vi "Validate.vi"(8 "error in (no error)":errorcluster, 9 "in build?":bool, 10 "proj refnum":refnum<vi>, 11 "IB_Source_Build in":refnum<class "IB_Source_Build.lvclass">) -> (0 "error out":errorcluster, 3 "IB_Source_Build out":refnum<class "IB_Source_Build.lvclass">)   [LabVIEW 2020, in "IB_Source_Build.lvclass"]
uses:
  <vilib>/AppBuilder/IB_Classes/Source/Container/Build/IB_Source_Build.lvclass
  <vilib>/AppBuilder/IB_Classes/Source/Container/Build/IB_Source_Build.lvclass/IB_Source_Build.ctl
  <vilib>/AppBuilder/IB_Classes/Source/IB_Source.lvclass
  <vilib>/AppBuilder/IB_Classes/Source/Container/IB_Source_Container.lvclass
  <vilib>/AppBuilder/IB_Classes/Source/File/CtrFile/IB_CtrFile.lvclass
  e:/builds/penguin/labview/branches/2020/dev/dist/vi.lib/AppBuilder/IB_Classes/Source/Container/IB_Source_Container.lvclass
  e:/builds/penguin/labview/branches/2020/dev/dist/vi.lib/AppBuilder/IB_Classes/Source/IB_Source.lvclass
  e:/builds/penguin/labview/branches/2020/dev/dist/vi.lib/AppBuilder/IB_Classes/Source/Container/Build/IB_Source_Build.lvclass
  e:/builds/penguin/labview/branches/2020/dev/dist/vi.lib/AppBuilder/IB_Classes/Source/File/IB_Source_File.lvclass
  e:/builds/penguin/labview/branches/2020/dev/dist/vi.lib/AppBuilder/IB_Classes/Source/File/CtrFile/IB_CtrFile.lvclass
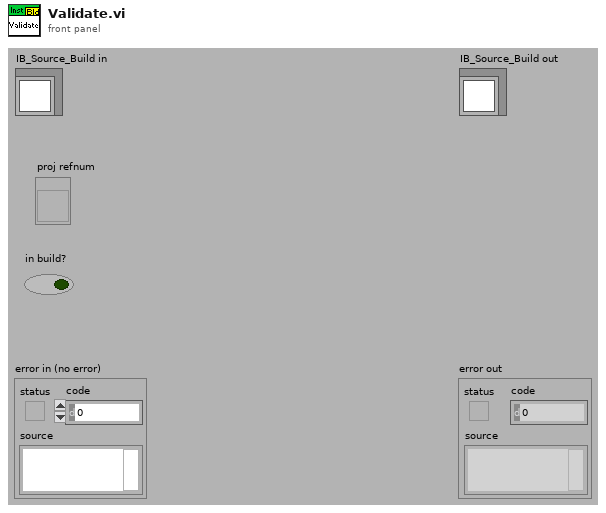
[diagram p1: front panel]
types:
  T1 = typedef "IB_Source_Container.ctl" = cluster{"files":refnum<class "IB_CtrFile.lvclass">[], "previewed?":bool, "preview error?":bool}
  T2 = typedef "IB_Source.ctl" = cluster{"name":string, "sourceTag":string, "destTag":string, "path":path, "eng_installPath":string, "UI_inBuild?":bool, "str ref?":bool}
  T3 = typedef "SRdB_Bld.ctl" = cluster{"ItemID":string, "FileItemIDs":string[], "RelPaths":string[], "AbsPaths":path[], "preview error?":bool, "Dependencies":T4[]}
  T4 = typedef "AB_Dependency.ctl" = cluster{"path":path, "delimited name":string, "type":T5}
  T5 = typedef "NI_FileType.lvlib/LVFileType.ctl" = enum32{"Invalid file", "Unknown type", "Instrument", "Control", "Polymorphic VI", "Project", "Library", "LVClass", "XControl", "XNode", "Shared library", ".NET assembly", "ActiveX interface", "CIN", "Run-time menu", "Palette menu", "Help file", "LLB", "XNode Edit Dependency", "Class Private Data Control", "Statechart", "MathScript .m file", "Ladder Diagram", "LVLibp", "XNode Build Dependency"}
  T6 = typedef "IB_CtrFile.ctl" = cluster{"parentTag":string, "force save?":bool}
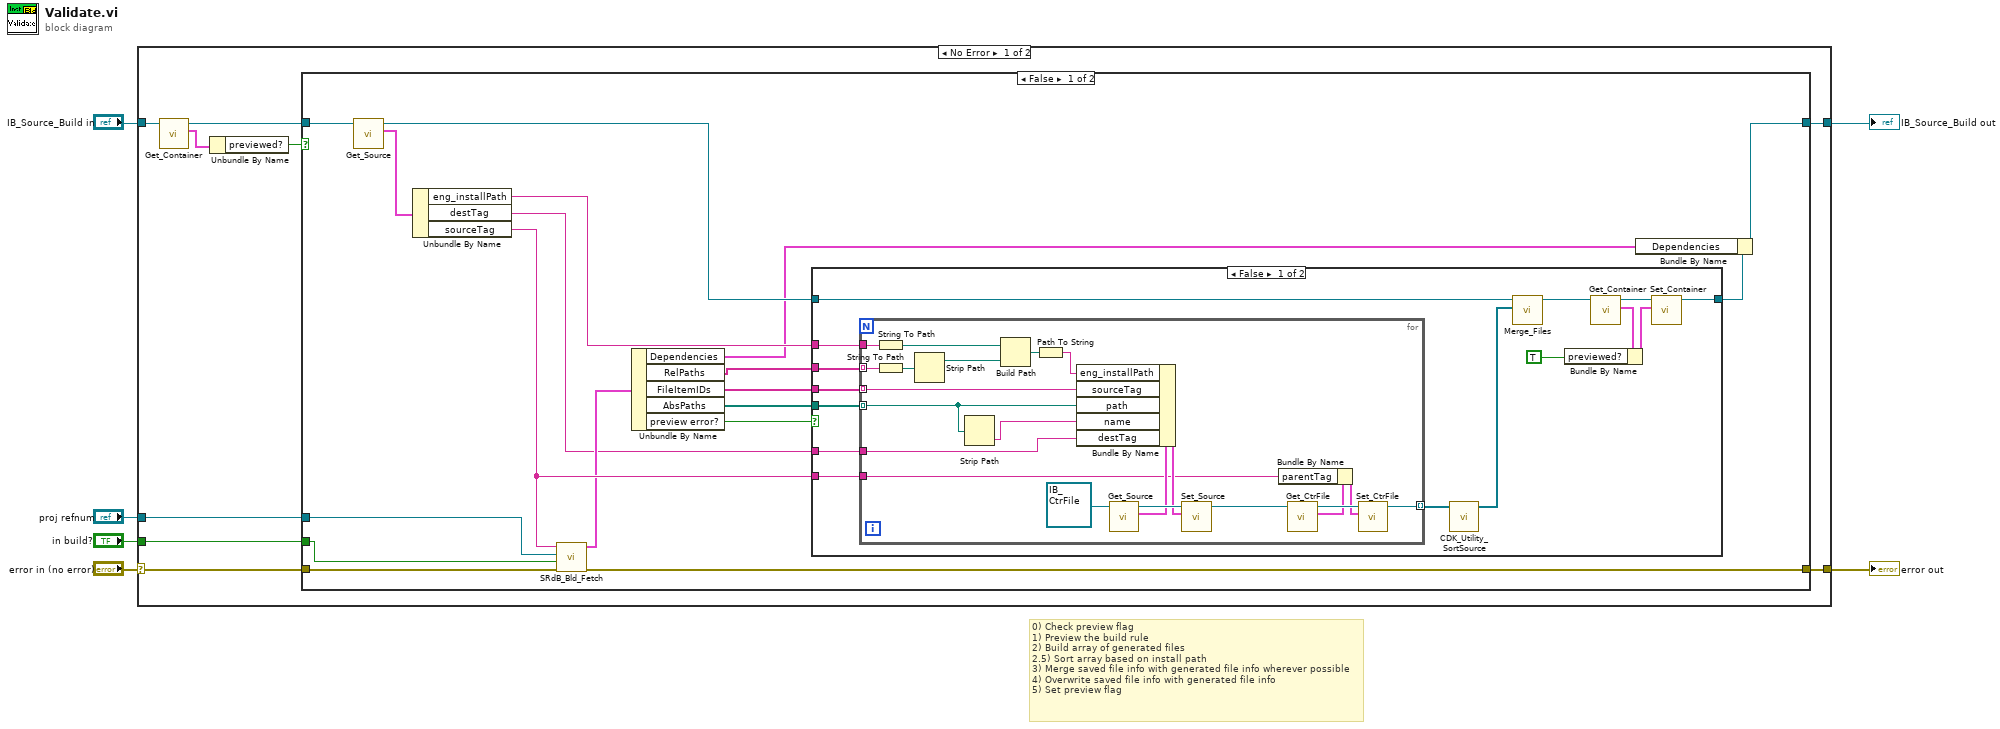
[diagram p0: block diagram]
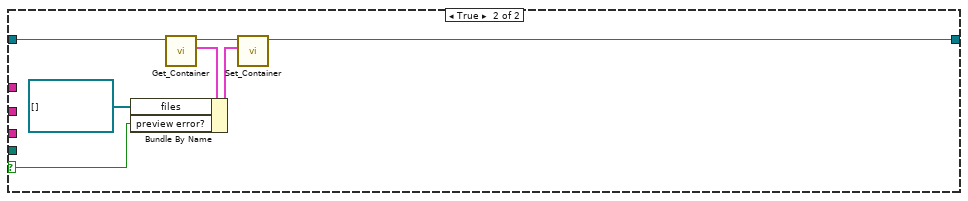
[diagram p2: hidden frame]
diagram:
  # "0) Check preview flag\n1) Preview the build rule\n2) Build array of generated files\n2.5) Sort array based on install path\n3) Merge saved file info with generated file info wherever possible\n4) Overwrite saved file info with generated file info\n5) Set preview flag"
  n1 = case shown="No Error" "error in (no error)" {
    selector: "error in (no error)" -> [w13 w80]
    tunnel: [w12 w80] -> w5
    tunnel: "IB_Source_Build in" -> [w10 w79]
    tunnel: "proj refnum" -> [w14 _]
    tunnel: [w15 w79] -> w2
    tunnel: "in build?" -> [w7 _]
    frame No Error {
      n2 = call <vilib>:"Get_Container.vi"("IB_Source_Container in"=w10) -> ("data"=w8:T1, "IB_Source_Container out"=w9:refnum<class "IB_Source_Build.lvclass">)  [unwired: 1 in, 8 out]
      n3 = Unbundle By Name(w8) -> ("previewed?"=w11:bool)
      n4 = case shown="False" w11 {
        tunnel: w9 -> [w21 w78]
        tunnel: [w18 w78] -> w15
        tunnel: w14 -> [w22 _]
        tunnel: w13 -> [w30 w77]
        tunnel: [w23 w77] -> w12
        tunnel: w7 -> [w19 _]
        frame False {
          n5 = call <vilib>:"Get_Source.vi"("IB_Source in"=w21) -> ("data"=w33:T2, "IB_Source out"=w24:refnum<class "IB_Source_Build.lvclass">)  [unwired: 1 in, 8 out]
          n6 = Unbundle By Name(w33) -> ("eng_installPath"=w32:string, "destTag"=w25:string, "sourceTag"=w31:string)
          n7 = call <resource>:"SRdB_Bld_Fetch.vi"("error in (no error)"=w30, "in build?"=w19, "Project"=w22, "itemID"=w31) -> ("error out"=w23:errorcluster, "build"=w29:T3)  [unwired: 6 out]
          n8 = Unbundle By Name(w29) -> ("Dependencies"=w16:T4[], "RelPaths"=w28:string[], "FileItemIDs"=w27:string[], "AbsPaths"=w26:path[], "preview error?"=w20:bool)
          n9 = case shown="False" w20 {
            selector: w20 -> [_ w70]
            tunnel: w32 -> [w48 _]
            tunnel: [w35 w72] -> w17
            tunnel: w31 -> [w45 _]
            tunnel: w28 -> [w44 _]
            tunnel: w27 -> [w43 _]
            tunnel: w26 -> [w42 _]
            tunnel: w25 -> [w41 _]
            tunnel: w24 -> [w40 w73]
            frame False {
              n10 = for {
                tunnel: w42 -> [w65] mode=indexing
                tunnel: w43 -> [w66] mode=indexing
                tunnel: [w54] -> w47 mode=indexing
                tunnel: w44 -> [w61] mode=indexing
                tunnel: w48 -> [w60]
                tunnel: w41 -> [w56]
                tunnel: w45 -> [w49]
                n11 = String To Path(string=w60) -> (path=w62:path)
                n12 = String To Path(string=w61) -> (path=w58:path)
                n13 = Strip Path(path=w58) -> (stripped path=w57:path)  [unwired: 1 out]
                n14 = Strip Path(path=w65) -> (name=w64:string)  [unwired: 1 out]
                n15 = Build Path(base path=w62, name or relative path=w57) -> (appended path=w63:path)
                n16 = Path To String(path=w63) -> (string=w59:string)
                n17 = call <vilib>:"Get_Source.vi"("IB_Source in"=refnum<class "IB_CtrFile.lvclass"> refnum ("IB_CtrFile.lvclass")) -> ("data"=w68:T2, "IB_Source out"=w69:refnum<class "IB_CtrFile.lvclass">)  [unwired: 1 in, 8 out]
                n18 = Bundle By Name(cluster=w68, "eng_installPath"=w59, "sourceTag"=w66, "path"=w65, "name"=w64, "destTag"=w56) -> (w67:T2)
                n19 = call <vilib>:"Set_Source.vi"("data"=w67, "IB_Source in"=w69) -> ("IB_Source out"=w53:refnum<class "IB_CtrFile.lvclass">)  [unwired: 1 in, 8 out]
                n20 = call <vilib>:"Get_CtrFile.vi"("IB_CtrFile in"=w53) -> ("parentTag"=w51:T6, "IB_CtrFile out"=w52:refnum<class "IB_CtrFile.lvclass">)  [unwired: 1 in, 8 out]
                n21 = Bundle By Name(cluster=w51, "parentTag"=w49) -> (w50:T6)
                n22 = call <vilib>:"Set_CtrFile.vi"("parentTag"=w50, "IB_CtrFile in"=w52) -> ("IB_CtrFile out"=w54:refnum<class "IB_CtrFile.lvclass">)  [unwired: 1 in, 8 out]
              }
              n23 = call <resource>:"CDK_Utility_SortSource.vi"("Source in"=w47) -> ("Source out"=w46:refnum<class "IB_CtrFile.lvclass">[])  [unwired: 10 out]
              n24 = call <vilib>:"Merge_Files.vi"("files"=w46, "IB_Source_Container in"=w40) -> ("IB_Source_Container out"=w36:refnum<class "IB_Source_Build.lvclass">)  [unwired: 2 in, 7 out]
              n25 = call <vilib>:"Get_Container.vi"("IB_Source_Container in"=w36) -> ("data"=w39:T1, "IB_Source_Container out"=w38:refnum<class "IB_Source_Build.lvclass">)  [unwired: 1 in, 8 out]
              n26 = Bundle By Name(cluster=w39, "previewed?"=TRUE) -> (w37:T1)
              n27 = call <vilib>:"Set_Container.vi"("data"=w37, "IB_Source_Container in"=w38) -> ("IB_Source_Container out"=w35:refnum<class "IB_Source_Build.lvclass">)  [unwired: 1 in, 8 out]
            }
            frame True {
              n28 = call <vilib>:"Get_Container.vi"("IB_Source_Container in"=w73) -> ("data"=w76:T1, "IB_Source_Container out"=w75:refnum<class "IB_Source_Build.lvclass">)  [unwired: 1 in, 8 out]
              n29 = Bundle By Name(cluster=w76, "files"=refnum<class "IB_CtrFile.lvclass">[] [], "preview error?"=w70) -> (w74:T1)
              n30 = call <vilib>:"Set_Container.vi"("data"=w74, "IB_Source_Container in"=w75) -> ("IB_Source_Container out"=w72:refnum<class "IB_Source_Build.lvclass">)  [unwired: 1 in, 8 out]
            }
          }
          n31 = Bundle By Name(cluster=w17, "Dependencies"=w16) -> (w18:refnum<class "IB_Source_Build.lvclass">)
        }
        frame True {
        }
      }
    }
    frame Error {
    }
  }
  "error out" <- w5
  "IB_Source_Build out" <- w2
